vi "OdorSeq_Main.vi"() -> ()   [LabVIEW 2016]
uses:
  <vilib>/event_ctls.llb/eventvkey.ctl
  Odour_component_data_GLOBAL.vi
  <vilib>/Utility/xml.llb/Read From XML File(string).vi
  Odour_stimuli.vi
  Odour_sequences.vi
  Odour component similarity map.vi
  Odour_protocol.vi
panel:
  in  "Tab Control":T1(tab)=enum."Stimuli"
  in  "Clear protocol":bool
  in  "Protocol cluster":T2={"Sequence"=[], "Rel. requency"=[5.0], "Frequency"=[5.0], "Sequence interval"=200.0, "Rarest sequence "=200.0, "Randomization"=2} {"Randomization" items=["None", "Simple shuffle", "Block"]; "Rarest sequence" format="%#_g /h"; "Sequence interval" format="%#_g ms"; "Frequency" format="%.3f"}
  in  "Save protocol":bool
  in  "Protocol":path
  in  "Sequences":i32(listbox)=7
  out "Stimulus similarity labels 2":string[](array[string])=["S1", "S2", "S3", "UNC S-", "UNC S+", "COND 1", "COND 2", "BLANK"]
  out "Stimulus similarity labels 1":string[](array[string])=["S1", "S2", "S3", "UNC S-", "UNC S+", "COND 1", "COND 2", "BLANK"]
  out "Stimulus similarity":u32[][](array[colorbox])=[[16711680, 5132031, 395007, 5921535, 255, 987135, 7434751, 255], [5132031, 16711680, 16775930, 16770276, 16760510, 16738922, 16767963, 255], [395007, 16775930, 16711680, 11382271, 16742777, 16776701, 12434943, 255], [5921535, 16770276, 11382271, 16723245, 16382463, 16772075, 16765136, 255], [255, 16760510, 16742777, 16382463, 16731726, 16740978, 12763903, 255], [987135, 16738922, 16776701, 16772075, 16740978, 16711680, 15000831, 255], [7434751, 16767963, 12434943, 16765136, 12763903, 15000831, 16724273, 255], [255, 255, 255, 255, 255, 255, 255, 16711680]]
  in  "Counter  13-16":i32(listbox)=-1
  in  "Counter  9-12":i32(listbox)=-1
  in  "Counter  5-8":i32(listbox)=-1
  in  "Trashcan":i32(listbox)
  in  "Stimuli":i32(listbox)=6
  in  "Stimulus properties":T3={"Name"="COND 2", "Bottles "=-1, "Conc."=10.0, "Unit"=enum."ppm", "Duration"=100.0, "Add stimulus button"=FALSE, "Remove stimulus button "=FALSE} {"Duration" format="%#_g ms"}
  in  "Counter  1-4":i32(listbox)=-1
  out "Color Box 21":u32(colorbox)=3381759
  out "Color Box 12":u32(colorbox)=9868950
  out "Color Box 12":u32(colorbox)
  out "Color Box 20":u32(colorbox)=15725235
  out "Color Box 19":u32(colorbox)=13140224
  out "Color Box 18":u32(colorbox)=8388736
  out "Color Box 17":u32(colorbox)=32896
  out "Color Box 16":u32(colorbox)=16711935
  out "Color Box 15":u32(colorbox)=8405056
  out "Color Box 14":u32(colorbox)=65535
  out "Color Box 13":u32(colorbox)=8388863
  out "Color Box 12":u32(colorbox)=16743025
  out "Color Box 11":u32(colorbox)=15990570
  out "Color Box 10":u32(colorbox)=255
  out "Color Box 9":u32(colorbox)=6618880
  out "Color Box 8":u32(colorbox)=16711680
  in  "Monomolecular":i32(listbox)=6
  in  "Mixture":i32(listbox)=2
  in  "Blank":i32(listbox)=2
  out "Bottle chemical similarity":cluster{"MDS1":dbl[], "MDS2":dbl[]}[](graph)=[{"MDS1"=[0.3189845978019478, -0.5958047359661698], "MDS2"=[-0.19587325078604045, -0.0928400576289578]}, {"MDS1"=[0.10987962122155093, -0.2773805044856591], "MDS2"=[-0.2505324334838407, -0.2170165090375375]}, {"MDS1"=[-0.6430615610179795, -0.10227449366179224], "MDS2"=[0.40234001920080187, -0.5044648362602937]}, {"MDS1"=[-0.4431658258870894, -0.024797457597433275], "MDS2"=[-0.29472177172362407, -0.49208323822896083]}, {"MDS1"=[0.4573556658647923], "MDS2"=[0.5384723425872284]}, {"MDS1"=[-0.17173498215634928], "MDS2"=[0.4360302310022115]}, {"MDS1"=[0.47823511863963886], "MDS2"=[0.3906686856455658]}, {"MDS1"=[-0.3589435679497024], "MDS2"=[0.4668292977954712]}, {"MDS1"=[-0.14564084129683338], "MDS2"=[0.2496266112085214]}, {"MDS1"=[0.47341517045736714], "MDS2"=[0.47574696538692657]}, {"MDS1"=[-0.6803573756720218], "MDS2"=[-0.439251267008941]}]
  in  "Sequence properties":T4={"Name"="COMPLEX 2D+", "Trigger"=2, "Stimulus interval"=10.0, "Add sequence button"=FALSE, "Remove sequence button "=FALSE, "Stimuli "=0, "Reward condition"=0} {"Reward condition" items=["None", "Both / middle", "Left", "Right", "No-go"]; "Trigger" items=["None", "Sequence start", "Each stimulus"]; "Stimulus interval" format="%#_6g ms"}
  in  "Color Box 2":u32(colorbox)=255
  in  "Color Box":u32(colorbox)=16711680
  in  "DistanceMatrixColorBox":u32[][](array[colorbox])=[[13158600, 13158600, 13158600, 13158600, 13158600, 13158600, 13158600, 13158600, 13158600, 13158600, 13158600, 13158600, 13158600, 13158600, 13158600, 13158600], [13158600, 16736609, 10461183, 255, 16053503, 12369151, 255, 255, 16764879, 255, 16771818, 16773874, 15987711, 255, 11382271, 5526783], [13158600, 10461183, 16711680, 255, 16769762, 16727871, 255, 255, 11974399, 255, 16774645, 16119295, 12303359, 255, 16711680, 1645055], [13158600, 255, 255, 16711680, 255, 255, 16711680, 16711680, 255, 16711680, 255, 255, 255, 16711680, 255, 255], [13158600, 16053503, 16769762, 255, 16711680, 16757426, 255, 255, 15724543, 255, 16766164, 16736095, 16750230, 255, 16763851, 2566143], [13158600, 12369151, 16727871, 255, 16757426, 16711680, 255, 255, 11645439, 255, 16771304, 16766678, 15987711, 255, 16716563, 255], [13158600, 255, 255, 16711680, 255, 255, 16711680, 16711680, 255, 16711680, 255, 255, 255, 16711680, 255, 255], [13158600, 255, 255, 16711680, 255, 255, 16711680, 16711680, 255, 16711680, 255, 255, 255, 16711680, 255, 255], [13158600, 16764879, 11974399, 255, 15724543, 11645439, 255, 255, 16734810, 255, 16760767, 16772075, 12698111, 255, 11842815, 7697919], [13158600, 255, 255, 16711680, 255, 255, 16711680, 16711680, 255, 16711680, 255, 255, 255, 16711680, 255, 255], [13158600, 16771818, 16774645, 255, 16766164, 16771304, 255, 255, 16760767, 255, 16731469, 16763080, 14606079, 255, 16772075, 6645247], [13158600, 16773874, 16119295, 255, 16736095, 16766678, 255, 255, 16772075, 255, 16763080, 16711680, 16758454, 255, 16773103, 5724159], [13158600, 15987711, 12303359, 255, 16750230, 15987711, 255, 255, 12698111, 255, 14606079, 16758454, 16711680, 255, 14013951, 1776639], [13158600, 255, 255, 16711680, 255, 255, 16711680, 16711680, 255, 16711680, 255, 255, 255, 16711680, 255, 255], [13158600, 11382271, 16711680, 255, 16763851, 16716563, 255, 255, 11842815, 255, 16772075, 16773103, 14013951, 255, 16711680, 855551], [13158600, 5526783, 1645055, 255, 2566143, 255, 255, 255, 7697919, 255, 6645247, 5724159, 1776639, 255, 855551, 16711680]]
  out "Odour bottles":T5(array[cluster])=[[{"Mixture components"=[{"Name"="Acetophenone", "CID"=8174, "Volatility"=0.45}, {"Name"="Fenchone", "CID"=8635, "Volatility"=0.82}], "Name"="B1 (ME1)", "VPs"="6.4E-1 ± 41%", "Proportion"=[{"Numeric"=50.0}, {"Numeric"=50.0}], "Selected"=TRUE}, {"Mixture components"=[{"Name"="Methyl benzoate", "CID"=8103, "Volatility"=0.38}, {"Name"="Menthone", "CID"=8063, "Volatility"=0.28}], "Name"="B2 (ME2)", "VPs"="3.3E-1 ± 21%", "Proportion"=[{"Numeric"=50.0}, {"Numeric"=50.0}], "Selected"=FALSE}, {"Mixture components"=[{"Name"="Decanol", "CID"=460, "Volatility"=0.00851}], "Name"="B3 (C4f)", "VPs"="8.5E-3", "Proportion"=[{"Numeric"=100.0}], "Selected"=FALSE}, {"Mixture components"=[{"Name"="MINERAL OIL", "CID"=0, "Volatility"=0.0}], "Name"="B4 (Bl)", "VPs"="0.0E+0", "Proportion"=[{"Numeric"=100.0}], "Selected"=FALSE}], [{"Mixture components"=[{"Name"="Heptanoic acid ", "CID"=957, "Volatility"=0.0107}], "Name"="B5 (C3cA)", "VPs"="1.1E-2", "Proportion"=[{"Numeric"=100.0}], "Selected"=FALSE}, {"Mixture components"=[{"Name"="Octanol", "CID"=7439, "Volatility"=0.0794}], "Name"="B6 (C4cA)", "VPs"="7.9E-2", "Proportion"=[{"Numeric"=100.0}], "Selected"=FALSE}, {"Mixture components"=[{"Name"="MINERAL OIL", "CID"=0, "Volatility"=0.0}], "Name"="B7 (Bl)", "VPs"="0.0E+0", "Proportion"=[{"Numeric"=100.0}], "Selected"=FALSE}, {"Mixture components"=[{"Name"="MINERAL OIL", "CID"=0, "Volatility"=0.0}], "Name"="B8 (Bl)", "VPs"="0.0E+0", "Proportion"=[{"Numeric"=100.0}], "Selected"=FALSE}], [{"Mixture components"=[{"Name"="Geranyl acetate", "CID"=6985, "Volatility"=0.03}, {"Name"="Dimethylacetophenone", "CID"=7144, "Volatility"=0.063}], "Name"="B9 (MW1)", "VPs"="4.6E-2 ± 50%", "Proportion"=[{"Numeric"=50.0}, {"Numeric"=50.0}], "Selected"=FALSE}, {"Mixture components"=[{"Name"="MINERAL OIL", "CID"=0, "Volatility"=0.0}], "Name"="B10 (Bl)", "VPs"="0.0E+0", "Proportion"=[{"Numeric"=100.0}], "Selected"=FALSE}, {"Mixture components"=[{"Name"="Geraniol", "CID"=6405, "Volatility"=0.03}, {"Name"="Phenyl butanone", "CID"=7762, "Volatility"=0.1}], "Name"="B11 (MW2)", "VPs"="6.5E-2 ± 76%", "Proportion"=[{"Numeric"=50.0}, {"Numeric"=50.0}], "Selected"=FALSE}, {"Mixture components"=[{"Name"="Pentyl acetate", "CID"=12348, "Volatility"=3.5}], "Name"="B12 (C3f)", "VPs"="3.5E+0", "Proportion"=[{"Numeric"=100.0}], "Selected"=FALSE}], [{"Mixture components"=[{"Name"="Valeric acid", "CID"=8025, "Volatility"=0.196}], "Name"="B13 (C3cB)", "VPs"="2.0E-1", "Proportion"=[{"Numeric"=100.0}], "Selected"=FALSE}, {"Mixture components"=[{"Name"="MINERAL OIL", "CID"=0, "Volatility"=0.0}], "Name"="B14 (Bl)", "VPs"="0.0E+0", "Proportion"=[{"Numeric"=100.0}], "Selected"=FALSE}, {"Mixture components"=[{"Name"="Nonanol", "CID"=4133, "Volatility"=0.0227}], "Name"="B15 (C4cB)", "VPs"="2.3E-2", "Proportion"=[{"Numeric"=100.0}], "Selected"=FALSE}, {"Mixture components"=[{"Name"="Hydroxacetophenone", "CID"=7462, "Volatility"=0.0856}], "Name"="B16 (Ol)", "VPs"="8.6E-2", "Proportion"=[{"Numeric"=100.0}], "Selected"=FALSE}]] {"Proportion"."Numeric" format="%d%%"}
  in  "Odour chemicals":i32(listbox)=36
  out "Chemical similarity":cluster{"MDS1":dbl[], "MDS2":dbl[]}[](graph)=[{"MDS1"=[], "MDS2"=[]}, {"MDS1"=[396.3821953927539, -262.41250467128555, -231.36430031040578, 114.07056457899871, -29.645616081049297, 58.40307821935197, -213.3415540440491, 252.76854811630145, 114.59724760685786, 12.179301078164926, 213.71781772180816, 10.245213827208765, -317.9647981045101, 249.27752347690375, -296.4544615523987, -26.698853099282278, -303.9529163482059, -23.502678410472118, -79.59753085274536, -76.44304440140283, -294.6567457719659, 112.29360419618213, -273.35122450752266, -294.76791641311274, -269.340230018179, -191.41524828002733, 251.79971870928094, 205.2249479165084, 515.3849497534994, -126.91499848915312, -152.14035558594634, -152.674775911407, -208.04948323720893, -111.19908951088753, -235.0545852465996, -236.20336645538308, -165.64242245257407, 110.87943807753645, -159.5151592759888, -148.46677914865614, 197.2464957982167, -232.541000525234, -187.82662250571298, -122.94463556800827, -191.8219737813257, 180.22600495656366, 51.353048668431704, -158.52742292807153, 266.82605746771884, -244.97562606669857, 207.17154717294608, -35.65469956598489, 256.9928159423369, -246.95298712232488, 143.47309690220376, -252.7110045881726, 150.23211981471368, 21.156685543603103, 179.59046460245207, -210.9178904519634, 281.28159545024744, 47.27018090750722, 185.8537823396016, -120.17144764398293, 119.41963149938562, -58.24361669961045, 17.20580648407221, -19.733594212360888, -2.8949993967070853, 14.89385579391006, 204.32713615045907, 31.18693554024182, 236.49773623152166, 37.27700380001177, 51.170561159934444, 297.4652966197888, 258.01381231117176, 93.81548252939837, 98.13934241781413, 233.76965217524653, 147.75453833538387, 339.8533239503384, -inf], "MDS2"=[-294.1625463085245, 75.06909387065261, 203.83961706757722, -243.76771476212969, -281.62183144789145, -228.79990905087422, 296.65536658552134, -250.34883594312083, -96.63812347643292, -164.80443024342875, -327.1617713637844, -277.3638544350568, -43.831335920252606, -213.31743810727397, 107.12891384196561, -87.93548942481429, 9.54512145075226, -253.81154308548392, -324.2771585204367, -273.6441237325548, 122.4114919562466, 39.85287306331019, -42.263086129371295, 191.0620800004279, -95.83774156123017, 142.3631394442883, -161.91563269564605, -308.24507263086724, -68.17744072149127, 102.91867516437394, -143.60083658864872, 243.13326408951488, -158.23331010430897, 208.56819115230442, -26.650521263465556, -104.36500693122969, -73.95049456240373, 170.98018005743705, 8.436616623045376, -213.0788157505672, -238.619079383165, 130.6588221918013, 101.29743735356698, 191.9015477463772, 189.9450263215761, 104.35598527492789, -178.40967800200966, -249.66981496564088, 13.479384089782926, -207.08642326769737, -174.93797693620664, 270.2139888611614, -68.61957940549138, -204.5270138088883, -211.27776405264314, -217.6654971930947, 221.1580180551867, -115.32895882976128, -56.04022976112759, 38.88407874545689, 102.71121558509061, -66.65120683967478, 288.33901581648973, 295.9933132570569, -28.685096728203234, 130.29205926060382, -8.697992950423888, 18.78620227069331, 37.62756232510908, 133.32677712624545, 160.28624069412643, 86.77073317156534, 93.65722557836662, 217.8007894783545, 191.40195381349582, 315.17787277483853, 146.47302969001294, 259.6981542624837, 398.7044129905194, 190.396254515234, 281.1287978570423, 251.5898534107341, -inf]}]
  in  "Distance metric":string(combo)="canberra_all"
  # "1"
  # "2"
  # "3"
  # "4"
  # "5"
  # "6"
  # "7"
  # "8"
  # "9"
  # "10"
  # "11"
  # "12"
  # "13"
  # "14"
  # "15"
  # "16"
  # "1"
  # "2"
  # "3"
  # "4"
  # "Similar"
  # "5"
  # "6"
  # "Different"
  # "7"
  # "8"
  # "9"
  # "10"
  # "11"
  # "12"
  # "13"
  # "14"
  # "15"
  # "16"
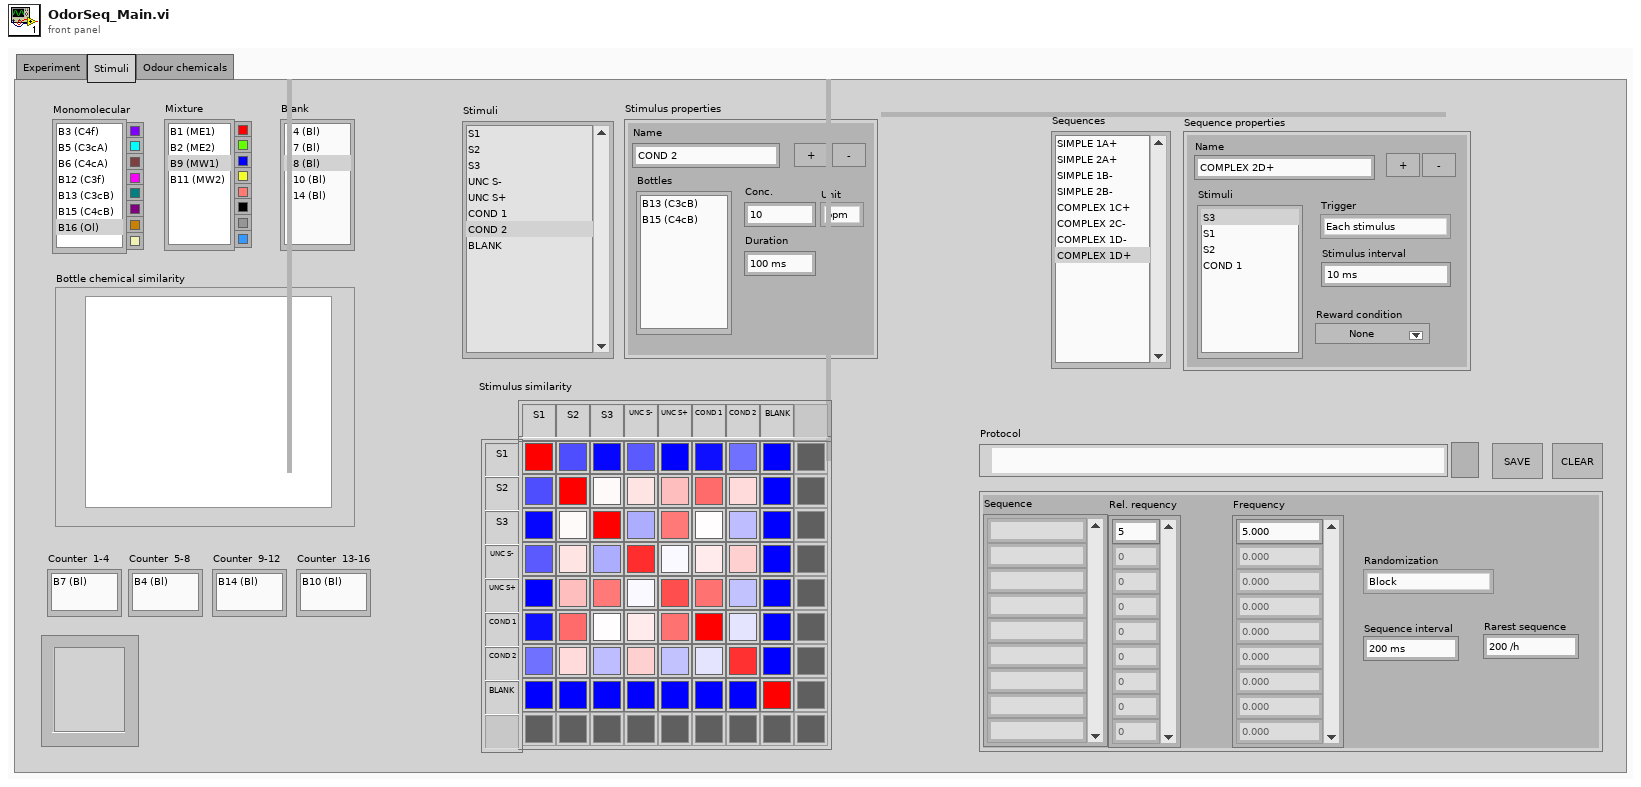
[diagram p1: front panel]
types:
  T1 = enum32{"Experiment", "Stimuli", "Odour chemicals"}
  T2 = cluster{"Sequence":string[], "Rel. requency":dbl[], "Frequency":dbl[], "Sequence interval":dbl, "Rarest sequence ":dbl, "Randomization":u16}
  T3 = cluster{"Name":string, "Bottles ":i32, "Conc.":dbl, "Unit":enum16{"%", "ppm"}, "Duration":dbl, "Add stimulus button":bool, "Remove stimulus button ":bool}
  T4 = cluster{"Name":string, "Trigger":u16, "Stimulus interval":dbl, "Add sequence button":bool, "Remove sequence button ":bool, "Stimuli ":i32, "Reward condition":u16}
  T5 = cluster{"Mixture components":cluster{"Name":string, "CID":i32, "Volatility":dbl}[], "Name":string, "VPs":string, "Proportion":cluster{"Numeric":dbl}[], "Selected":bool}[][]
  T6 = cluster{"names":string[], "CID":i32[], "volatility":dbl[], "2D map":dbl[][], "distance matrix":dbl[][]}
  T7 = cluster{"Name":string, "Bottles":i32[], "Conc.":dbl, "Unit":enum16{"%", "ppm"}, "Frequency":dbl}[]
  T8 = cluster{"Name":string, "Trigger":u16, "Stimulus interval":dbl, "Stimuli":i32[], "Reward condition":u16}[]
  T9 = cluster{"Name":string, "Bottles":i32[], "Conc.":dbl, "Unit":enum16{"%", "ppm"}, "Frequency":dbl}
  T10 = cluster{"Name":string, "Trigger":u16, "Stimulus interval":dbl, "Stimuli":i32[], "Reward condition":u16}
  T11 = typedef "eventvkey.ctl" = enum16{"ASCII", "Enter", "Return", "Shift", "Ctrl", "Alt", "Cmd", "Opt", "Caps", "NumLock", "Clear", "Break", "Up", "Down", "Left", "Right", "Insert", "Delete", "Home", "End", "PageUp", "PageDown", "Escape", "Help", "Pause", "ScrollLock", "F1", "F2", "F3", "F4", "F5", "F6", "F7", "F8", "F9", "F10", "F11", "F12", "F13", "F14", "F15", "F16", "F17", "F18", "F19", "F20", "F21", "F22", "F23", "F24", "Play", "VolumeUp", "VolumeDown", "Mute", "Two Byte Char"}
  T12 = cluster{"names":string[], "CID":i32[], "Vapour pressure":dbl[], "2D map":dbl[][], "distance matrix":dbl[][]}
  T13 = cluster{"Mixture components":cluster{"Name":string, "CID":i32, "Volatility":dbl}[], "Name":string, "VPs":string, "Proportion":cluster{"Numeric":dbl}[], "Selected":bool}[]
  T14 = cluster{"Name":string, "CID":i32, "Volatility":dbl}[]
  T15 = typedef "LVPoint32TypeDef.ctl" = cluster{"Horizontal":i32, "Vertical":i32}
  T16 = typedef "LVBoundsTypeDef.ctl" = cluster{"Width":u32, "Height":u32}
  T17 = typedef "LVPositionTypeDef.ctl" = cluster{"Left":i32, "Top":i32}
  T18 = cluster{"Mixture components":cluster{"Name":string, "CID":i32, "Volatility":dbl}[], "Name":string, "VPs":string, "Proportion":cluster{"Numeric":dbl}[], "Selected":bool}
  T19 = cluster{"Name":string, "Bottles":i32[], "Conc.":dbl, "Unit":enum16{"%", "ppm"}, "Duration":dbl}[]
  T20 = cluster{"Name":string, "Bottles":i32[], "Conc.":dbl, "Unit":enum16{"%", "ppm"}, "Duration":dbl}
  T21 = cluster{"data name":string, "drag data":variant}[]
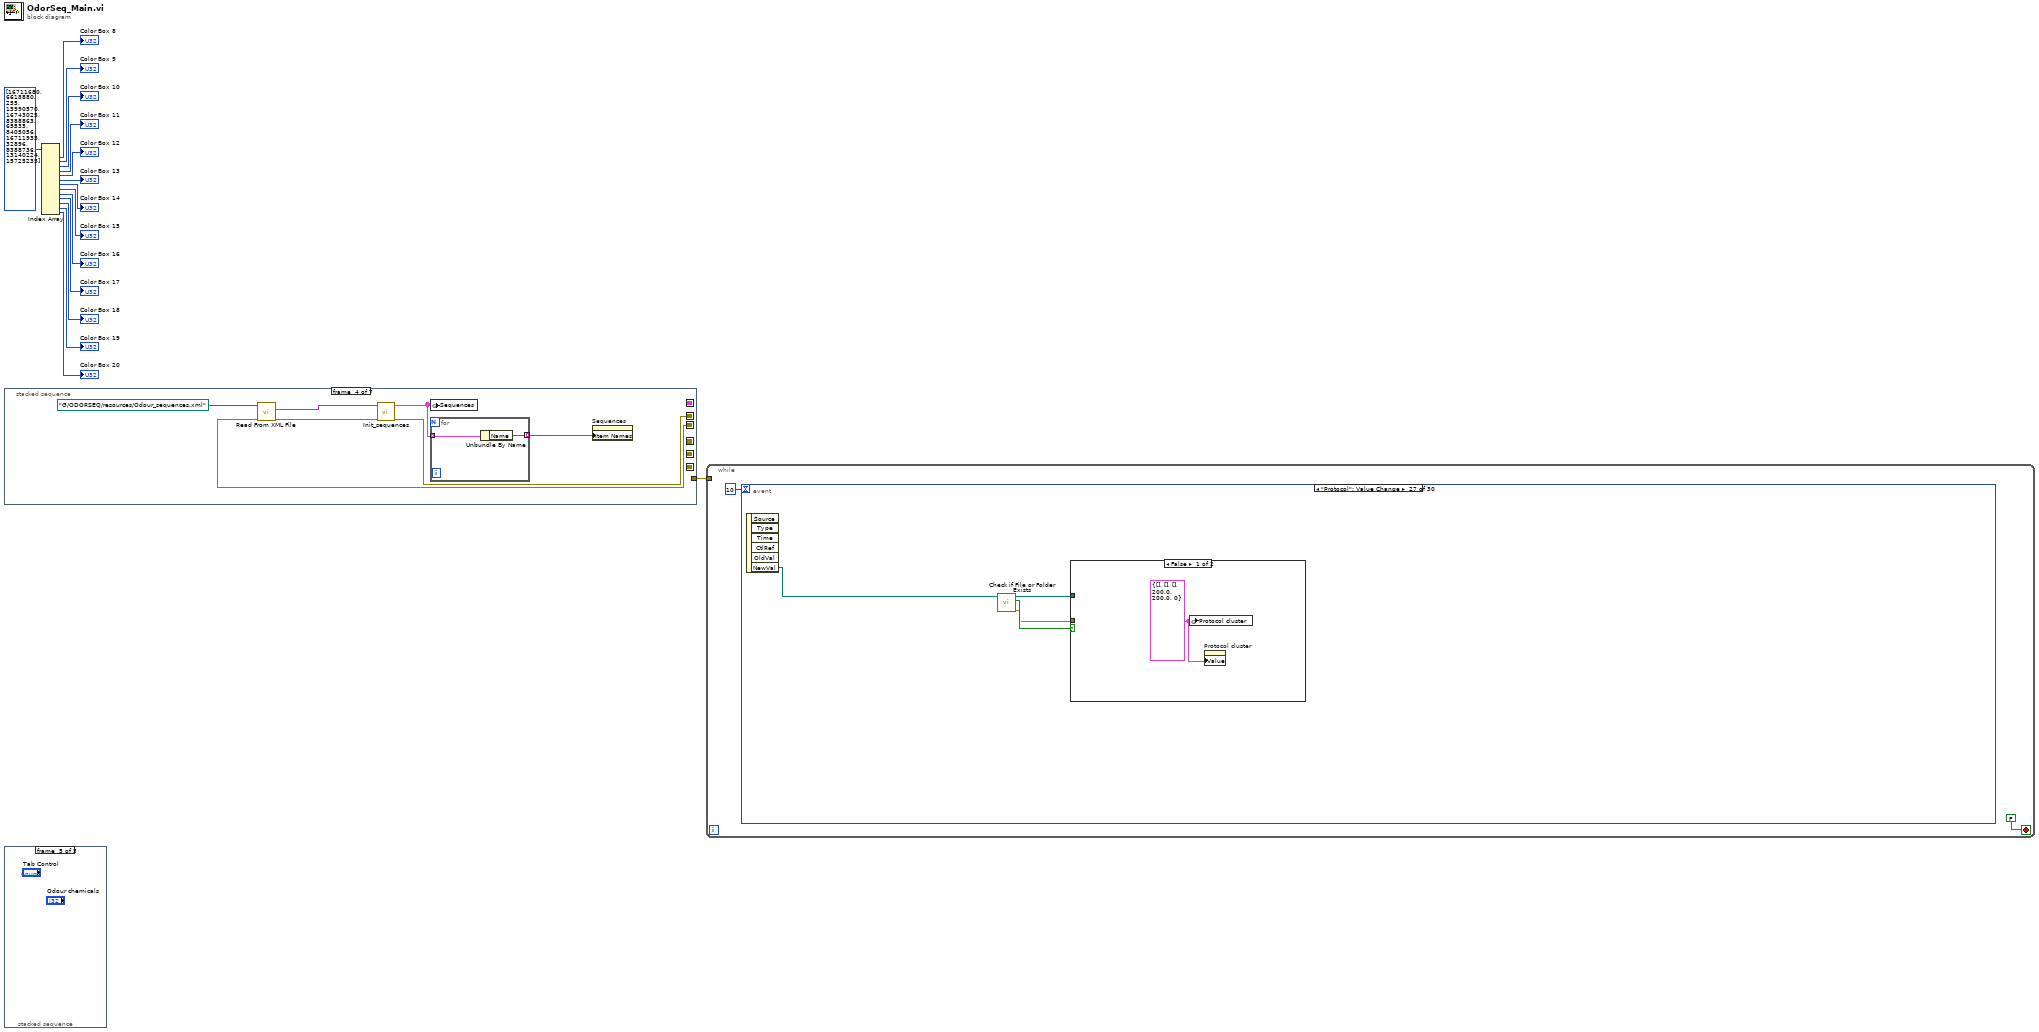
[diagram p0: block diagram]
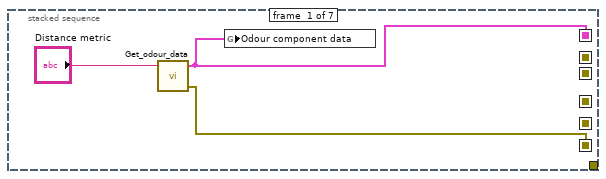
[diagram p2: hidden frame]
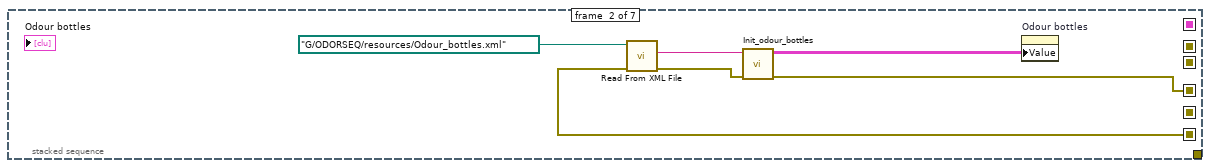
[diagram p3: hidden frame]
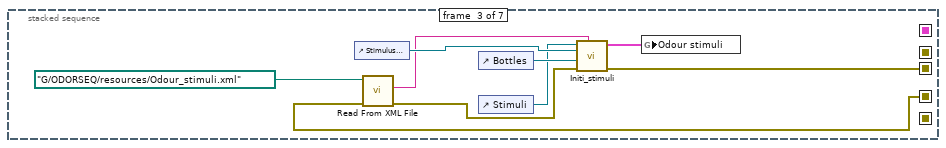
[diagram p4: hidden frame]
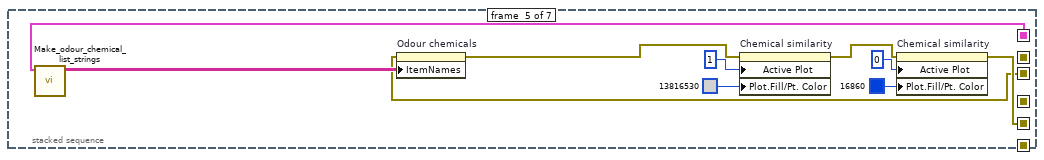
[diagram p5: hidden frame]
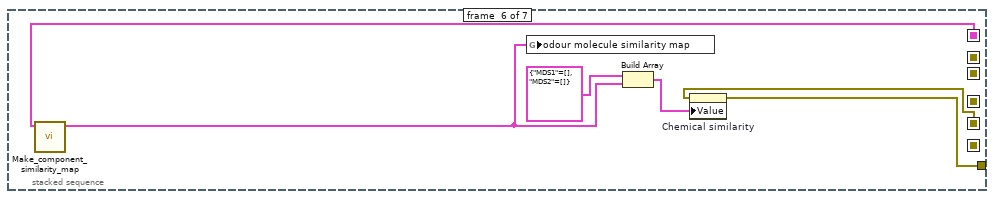
[diagram p6: hidden frame]
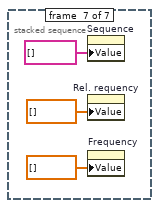
[diagram p7: hidden frame]
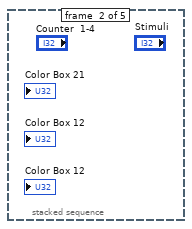
[diagram p9: hidden frame]
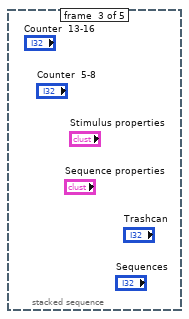
[diagram p10: hidden frame]
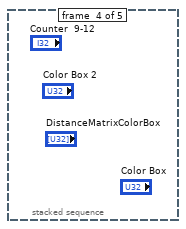
[diagram p11: hidden frame]
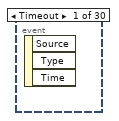
[diagram p12: hidden frame]
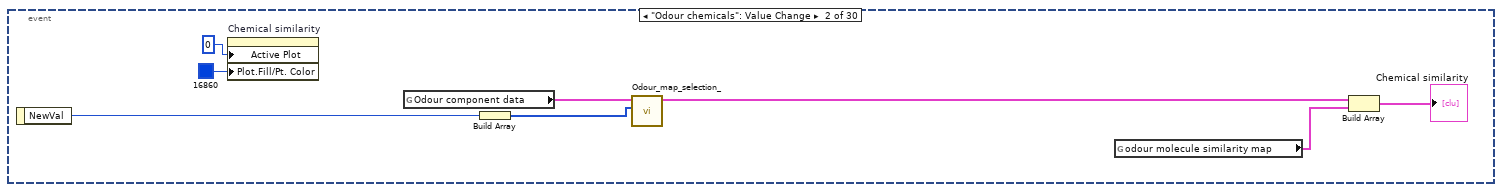
[diagram p13: hidden frame]
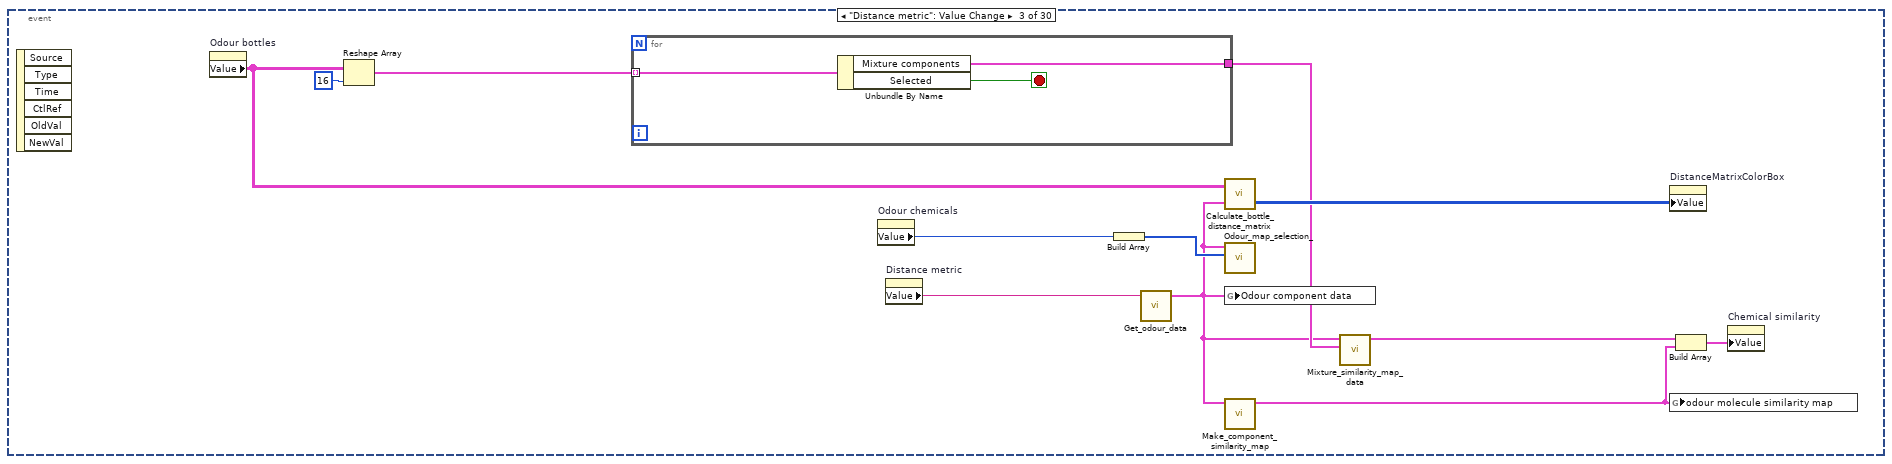
[diagram p14: hidden frame]
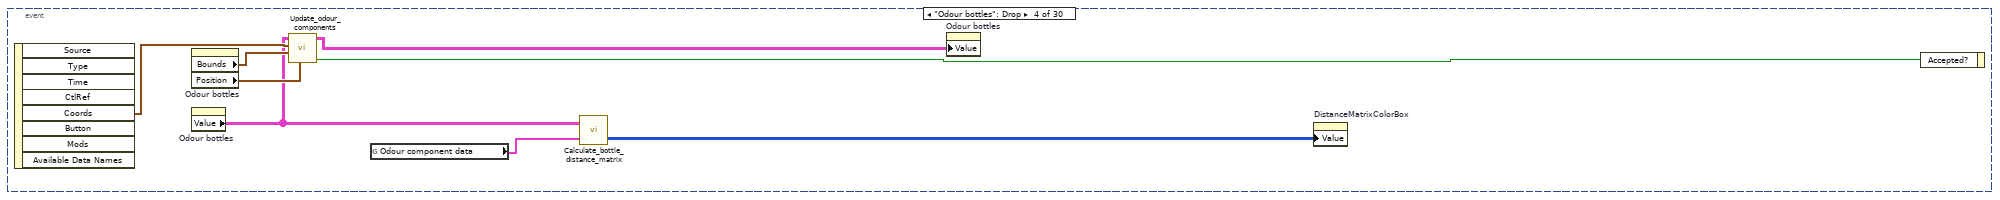
[diagram p15: hidden frame]
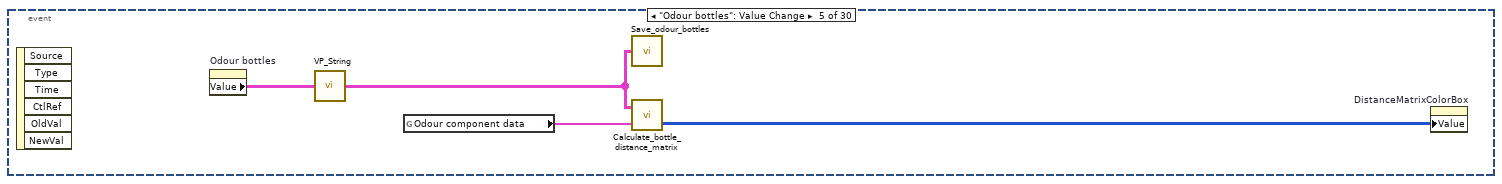
[diagram p16: hidden frame]
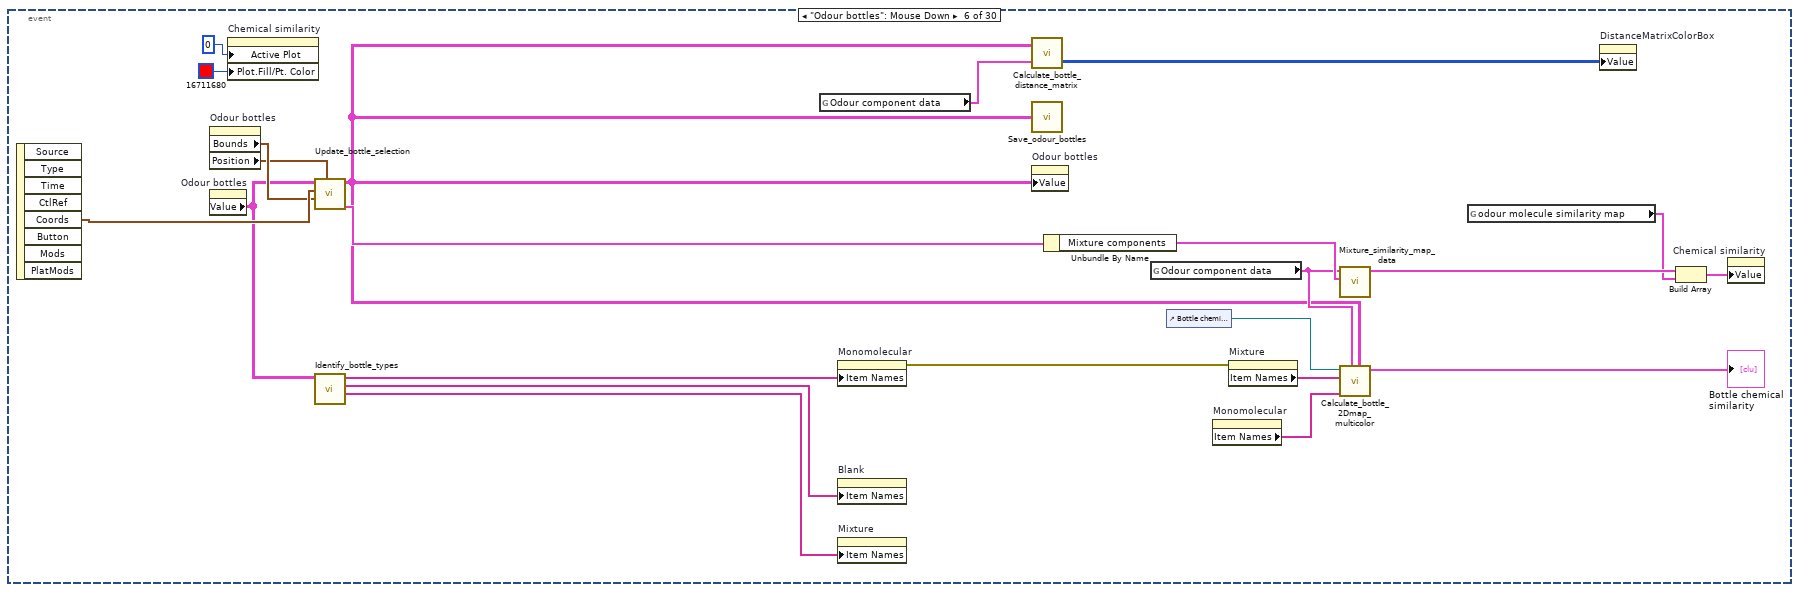
[diagram p17: hidden frame]
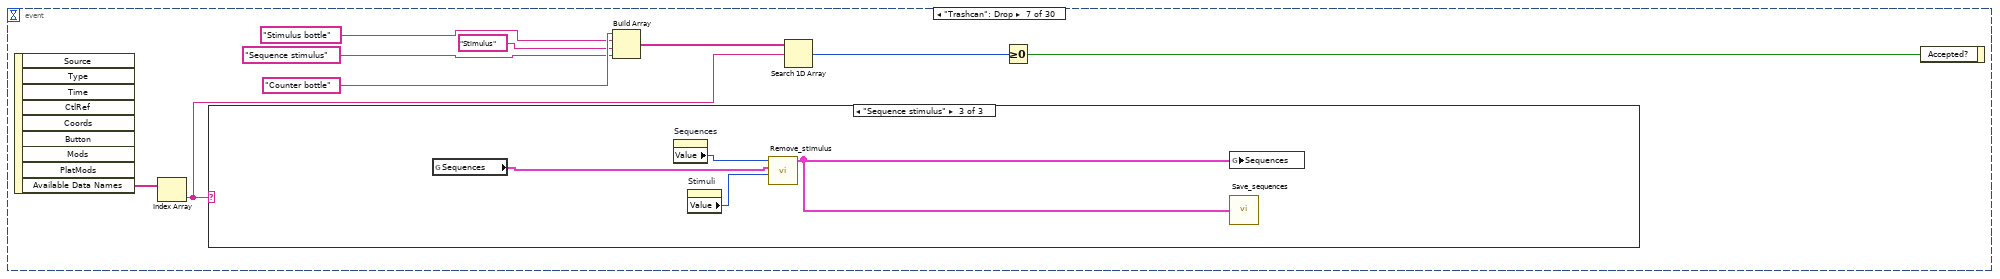
[diagram p18: hidden frame]
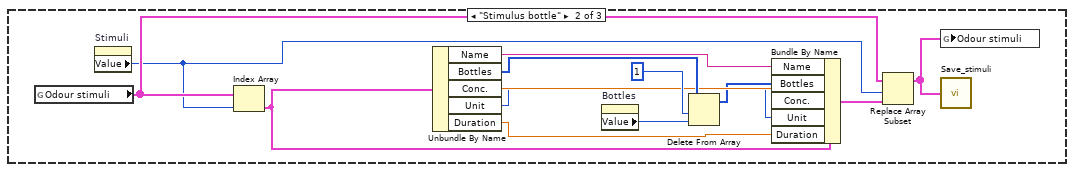
[diagram p20: hidden frame]
diagram:
  n1 = stacked-sequence {
    seq-local: [w16 _ _ _ _ _ _] -> [_ _ _ _ w44 w55 _]
    seq-local: [w17 _ _ _ _ _ _] -> [_ w21 _ _ _ _ _]
    seq-local: [_ w20 _ _ _ _ _] -> [_ _ w27 _ _ _ _]
    seq-local: [_ _ w26 _ _ _ _] -> [_ _ _ w40 w43 _ _]
    seq-local: [_ _ _ _ w45 _ _] -> [_ _ _ _ _ w54 _]
    seq-local: [_ _ _ w36 _ _ _] -> [_ _ _ _ _ _ _]
    tunnel: [_ _ _ _ _ w53 _] -> w1
    frame #0 {
      n2 = call "Get_odour_data.vi"("Distance metric"="Distance metric") -> ("error out"=w17:errorcluster, "Odour component data"=w16:T6)  [unwired: 3 in]
      n3 = global write "Odour_component_data_GLOBAL.vi" "Odour component data"(w16) -> ()
    }
    frame #1 {
      n4 = call-poly <vilib>:"Read From XML File.vi"("error in (no error)"=w21, "XML File Path"=path "G:/ODORSEQ/resources/Odour_bottles.xml") -> ("error out"=w24:errorcluster, "XML Elements"=w23:string)  [unwired: 7 in, 1 out]
      n5 = call "Init_odour_bottles.vi"("error in (no error)"=w24, "XML Elements"=w23) -> ("error IO"=w20:errorcluster, "Array"=w19:T5)  [unwired: 8 in]
      n6 = property on="Odour bottles" class="Arr (strict)"("Value"=w19) -> ()  [unwired: 2 in, 2 out]
    }
    frame #2 {
      n7 = control-ref of="Stimulus properties"() -> (w32:refnum<vi>)
      n8 = call-poly <vilib>:"Read From XML File.vi"("error in (no error)"=w27, "XML File Path"=path "G:/ODORSEQ/resources/Odour_stimuli.xml") -> ("error out"=w28:errorcluster, "XML Elements"=w29:string)  [unwired: 7 in, 1 out]
      n9 = control-ref of="Bottles"() -> (w33:refnum<vi>)
      n10 = control-ref of="Stimuli"() -> (w31:refnum<vi>)
      n11 = call "Initi_stimuli.vi"("XML Elements"=w29, "error in (no error)"=w28, "LstBox Refnum in"=w33, "Clust Refnum"=w32, "ListBox in"=w31) -> ("error IO"=w26:errorcluster, "Array"=w25:T7)  [unwired: 5 in]
      n12 = global write "Odour_stimuli.vi" "Odour stimuli"(w25) -> ()
    }
    frame #3 {
      n13 = call-poly <vilib>:"Read From XML File.vi"("error in (no error)"=w40, "XML File Path"=path "G:/ODORSEQ/resources/Odour_sequences.xml") -> ("error out"=w37:errorcluster, "XML Elements"=w38:string)  [unwired: 7 in, 1 out]
      n14 = call "Init_sequences.vi"("error in (no error)"=w37, "XML Elements"=w38) -> ("error IO"=w36:errorcluster, "Sequences"=w34:T8)  [unwired: 8 in]
      n15 = global write "Odour_sequences.vi" "Sequences"(w34) -> ()
      n16 = for {
        tunnel: [w42] -> w35 mode=indexing
        tunnel: w34 -> [w41] mode=indexing
        n17 = Unbundle By Name(w41) -> ("Name"=w42:string)
      }
      n18 = property on="Sequences" class="LstBox (strict)"("Item Names"=w35) -> ()  [unwired: 2 in, 2 out]
    }
    frame #4 {
      n19 = call "Make_odour_chemical_list_strings.vi"("Odour component data"=w44) -> ("Array"=w51:string[][])  [unwired: 10 in]
      n20 = property on="Odour chemicals" class="MCListbox (strict)"(error in=w43, "ItemNames"=w51) -> (error out=w52:errorcluster)  [unwired: 1 in, 1 out]
      n21 = property on="Chemical similarity" class="XYGraph (strict)"(error in=w52, "Active Plot"=u32 1, "Plot.Fill/Pt. Color"=u32 13816530) -> (error out=w47:errorcluster)  [unwired: 1 in, 1 out]
      n22 = property on="Chemical similarity" class="XYGraph (strict)"(error in=w47, "Active Plot"=u32 0 ("Plot.Fill/Point Color"), "Plot.Fill/Pt. Color"=u32 16860) -> (error out=w45:errorcluster)  [unwired: 1 in, 1 out]
    }
    frame #5 {
      n23 = call "Make_component_similarity_map.vi"("Odour component data"=w55) -> ("input cluster"=w56:cluster{"MDS1":dbl[], "MDS2":dbl[]})  [unwired: 10 in]
      n24 = global write "Odour component similarity map.vi" "odour molecule similarity map"(w56) -> ()
      n25 = Build Array(cluster{"MDS1":dbl[], "MDS2":dbl[]} {"MDS1"=[], "MDS2"=[]} ("element"), w56) -> (w57:cluster{"MDS1":dbl[], "MDS2":dbl[]}[])
      n26 = property on="Chemical similarity" class="XYGraph (strict)"(error in=w54, "Value"=w57) -> (error out=w53:errorcluster)  [unwired: 1 in, 1 out]
    }
    frame #6 {
      n27 = property on="Sequence" class="Arr (strict)"("Value"=string[] [] ("Item Names")) -> ()  [unwired: 2 in, 2 out]
      n28 = property on="Rel. requency" class="Arr (strict)"("Value"=dbl[] [] ("Rel. requency")) -> ()  [unwired: 2 in, 2 out]
      n29 = property on="Frequency" class="Arr (strict)"("Value"=dbl[] [] ("Frequency")) -> ()  [unwired: 2 in, 2 out]
    }
  }
  n30 = stacked-sequence {
    frame #0 {
    }
    frame #1 {
    }
    frame #2 {
    }
    frame #3 {
    }
    frame #4 {
    }
  }
  n31 = Index Array(array=u32[] [16711680, 6618880, 255, 15990570, 16743025, 8388863, 65535, 8405056, 16711935, 32896, 8388736, 13140224, 15725235]) -> (element #1=→"Color Box 8":u32, element #2=→"Color Box 9":u32, element #3=→"Color Box 10":u32, element #4=→"Color Box 11":u32, element #5=→"Color Box 12":u32, element #6=→"Color Box 13":u32, element #7=→"Color Box 14":u32, element #8=→"Color Box 15":u32, element #9=→"Color Box 16":u32, element #10=→"Color Box 17":u32, element #11=→"Color Box 18":u32, element #12=→"Color Box 19":u32, element #13=→"Color Box 20":u32)  [unwired: 13 in]
  n32 = while {
    tunnel: w1 -> [_]
    stop <- FALSE stop-if-true
    n33 = event shown="[26] \"Protocol\": Value Change" {
      selector: _ -> [_ _ _ _ _ _ _ _ _ _ _ _ _ _ _ _ _ _ _ _ _ _ _ _ _ _ _ _ _ _]
      dyn-events: _ -> [_ _ _ _ _ _ _ _ _ _ _ _ _ _ _ _ _ _ _ _ _ _ _ _ _ _ _ _ _ _]
      timeout: 10 -> [_ _ _ _ _ _ _ _ _ _ _ _ _ _ _ _ _ _ _ _ _ _ _ _ _ _ _ _ _ _]
      event Timeout {
        n34 = event-data() -> ()  [unwired: 1 in, 3 out]
      }
      event "Odour chemicals": Value Change {
        n35 = event-data() -> ("NewVal"=w71:i32)  [unwired: 1 in]
        n36 = property on="Chemical similarity" class="XYGraph (strict)"("Active Plot"=u32 0 ("Plot.Fill/Point Color"), "Plot.Fill/Pt. Color"=u32 16860) -> ()  [unwired: 2 in, 2 out]
        n37 = global read "Odour_component_data_GLOBAL.vi" "Odour component data"() -> (w66:T12)
        n38 = Build Array(w71) -> (w65:i32[])
        n39 = call "Odour_map_selection_.vi"("Array"=w65, "Odour component data"=w66) -> ("input cluster"=w69:cluster{"MDS1":dbl[], "MDS2":dbl[]})  [unwired: 9 in]
        n40 = global read "Odour component similarity map.vi" "odour molecule similarity map"() -> (w64:cluster{"MDS1":dbl[], "MDS2":dbl[]})
        n41 = Build Array(w69, w64) -> (→"Chemical similarity":cluster{"MDS1":dbl[], "MDS2":dbl[]}[])
      }
      event "Distance metric": Value Change {
        n42 = event-data() -> ()  [unwired: 1 in, 6 out]
        n43 = property on="Odour bottles" class="Arr (strict)"() -> ("Value"=w77:T5)  [unwired: 2 in, 2 out]
        n44 = Reshape Array(w77, 16 ("dimension size")) -> (w76:T13)
        n45 = for {
          tunnel: w76 -> [w86] mode=indexing
          tunnel: [w84] -> w74
          stop <- w85 stop-if-true
          n46 = Unbundle By Name(w86) -> ("Mixture components"=w84:T14, "Selected"=w85:bool)
        }
        n47 = property on="Odour chemicals" class="MCListbox (strict)"() -> ("Value"=w81:i32)  [unwired: 2 in, 2 out]
        n48 = property on="Distance metric" class="CmbBox"() -> ("Value"=w80:string)  [unwired: 2 in, 2 out]
        n49 = Build Array(w81) -> (w83:i32[])
        n50 = call "Get_odour_data.vi"("Distance metric"=w80) -> ("Odour component data"=w72:T6)  [unwired: 3 in, 1 out]
        n51 = call "Calculate_bottle_distance_matrix.vi"("Odour component data"=w72, "Odour bottles"=w77) -> ("Colour grid"=w78:u32[][])  [unwired: 1 in]
        n52 = call "Odour_map_selection_.vi"("Array"=w83, "Odour component data"=w72) -> ()  [unwired: 9 in, 1 out]
        n53 = global write "Odour_component_data_GLOBAL.vi" "Odour component data"(w72) -> ()
        n54 = call "Make_component_similarity_map.vi"("Odour component data"=w72) -> ("input cluster"=w79:cluster{"MDS1":dbl[], "MDS2":dbl[]})  [unwired: 10 in]
        n55 = call "Mixture_similarity_map_data.vi"("Mixture components"=w74, "Odour component data"=w72) -> ("input cluster"=w73:cluster{"MDS1":dbl[], "MDS2":dbl[]})  [unwired: 9 in]
        n56 = property on="DistanceMatrixColorBox" class="Arr (strict)"("Value"=w78) -> ()  [unwired: 2 in, 2 out]
        n57 = global write "Odour component similarity map.vi" "odour molecule similarity map"(w79) -> ()
        n58 = Build Array(w73, w79) -> (w82:cluster{"MDS1":dbl[], "MDS2":dbl[]}[])
        n59 = property on="Chemical similarity" class="XYGraph (strict)"("Value"=w82) -> ()  [unwired: 2 in, 2 out]
      }
      event "Odour bottles": Drop {
        n60 = event-data() -> ("Coords"=w94:T15)  [unwired: 1 in, 7 out]
        n61 = property on="Odour bottles" class="Arr (strict)"() -> ("Bounds"=w92:T16, "Position"=w93:T17)  [unwired: 2 in, 2 out]
        n62 = property on="Odour bottles" class="Arr (strict)"() -> ("Value"=w88:T5)  [unwired: 2 in, 2 out]
        n63 = call "Update_odour_components.vi"("Position"=w93, "Bounds"=w92, "Coords"=w94, "Odour bottles in"=w88) -> ("accept"=w91:bool, "Odou bottle out"=w89:T5)  [unwired: 6 in]
        n64 = global read "Odour_component_data_GLOBAL.vi" "Odour component data"() -> (w87:T12)
        n65 = call "Calculate_bottle_distance_matrix.vi"("Odour component data"=w87, "Odour bottles"=w88) -> ("Colour grid"=w90:u32[][])  [unwired: 1 in]
        n66 = property on="Odour bottles" class="Arr (strict)"("Value"=w89) -> ()  [unwired: 2 in, 2 out]
        n67 = property on="DistanceMatrixColorBox" class="Arr (strict)"("Value"=w90) -> ()  [unwired: 2 in, 2 out]
        n68 = event-data("Accepted?"=w91) -> ()  [unwired: 1 in, 1 out]
      }
      event "Odour bottles": Value Change {
        n69 = event-data() -> ()  [unwired: 1 in, 6 out]
        n70 = property on="Odour bottles" class="Arr (strict)"() -> ("Value"=w97:T5)  [unwired: 2 in, 2 out]
        n71 = call "VP_String.vi"("Odour bottles"=w97) -> ("Odour bottles 2"=w95:T5)
        n72 = global read "Odour_component_data_GLOBAL.vi" "Odour component data"() -> (w96:T12)
        n73 = call "Save_odour_bottles.vi"("Odour bottles"=w95) -> ()
        n74 = call "Calculate_bottle_distance_matrix.vi"("Odour component data"=w96, "Odour bottles"=w95) -> ("Colour grid"=w98:u32[][])  [unwired: 1 in]
        n75 = property on="DistanceMatrixColorBox" class="Arr (strict)"("Value"=w98) -> ()  [unwired: 2 in, 2 out]
      }
      event "Odour bottles": Mouse Down {
        n76 = event-data() -> ("Coords"=w121:T15)  [unwired: 1 in, 7 out]
        n77 = property on="Odour bottles" class="Arr (strict)"() -> ("Bounds"=w120:T16, "Position"=w119:T17)  [unwired: 2 in, 2 out]
        n78 = property on="Odour bottles" class="Arr (strict)"() -> ("Value"=w106:T5)  [unwired: 2 in, 2 out]
        n79 = property on="Chemical similarity" class="XYGraph (strict)"("Active Plot"=u32 0 ("Plot.Fill/Point Color"), "Plot.Fill/Pt. Color"=u32 16711680) -> ()  [unwired: 2 in, 2 out]
        n80 = call "Update_bottle_selection.vi"("Position"=w119, "Bounds"=w120, "Coords"=w121, "Odour bottles in"=w106) -> ("selected bottle"=w105:T18, "Odour bottles out"=w99:T5)  [unwired: 4 in]
        n81 = call "Identify_bottle_types.vi"("Odour bottles"=w106) -> ("Mixture bottles"=w112:string[], "Blank bottles"=w114:string[], "Monomolecular bottles"=w113:string[])  [unwired: 8 in]
        n82 = global read "Odour_component_data_GLOBAL.vi" "Odour component data"() -> (w100:T12)
        n83 = property on="Monomolecular" class="LstBox (strict)"("Item Names"=w113) -> (error out=w103:errorcluster)  [unwired: 2 in, 1 out]
        n84 = property on="Blank" class="LstBox (strict)"("Item Names"=w114) -> ()  [unwired: 2 in, 2 out]
        n85 = property on="Mixture" class="LstBox (strict)"("Item Names"=w112) -> ()  [unwired: 2 in, 2 out]
        n86 = call "Calculate_bottle_distance_matrix.vi"("Odour component data"=w100, "Odour bottles"=w99) -> ("Colour grid"=w101:u32[][])  [unwired: 1 in]
        n87 = call "Save_odour_bottles.vi"("Odour bottles"=w99) -> ()
        n88 = property on="Odour bottles" class="Arr (strict)"("Value"=w99) -> ()  [unwired: 2 in, 2 out]
        n89 = Unbundle By Name(w105) -> ("Mixture components"=w104:T14)
        n90 = global read "Odour_component_data_GLOBAL.vi" "Odour component data"() -> (w102:T12)
        n91 = control-ref of="Bottle chemical similarity"() -> (w109:refnum<vi>)
        n92 = property on="Monomolecular" class="LstBox (strict)"() -> ("Item Names"=w108:string[])  [unwired: 2 in, 2 out]
        n93 = property on="Mixture" class="LstBox (strict)"(error in=w103) -> ("Item Names"=w111:string[])  [unwired: 1 in, 2 out]
        n94 = call "Mixture_similarity_map_data.vi"("Mixture components"=w104, "Odour component data"=w102) -> ("input cluster"=w118:cluster{"MDS1":dbl[], "MDS2":dbl[]})  [unwired: 9 in]
        n95 = call "Calculate_bottle_2Dmap_multicolor.vi"("XYGraph in"=w109, "Mixture"=w111, "Monomolecular"=w108, "Odour component data"=w102, "Odour bottles in"=w99) -> ("appended array"=→"Bottle chemical similarity":cluster{"MDS1":dbl[], "MDS2":dbl[]}[])  [unwired: 5 in]
        n96 = global read "Odour component similarity map.vi" "odour molecule similarity map"() -> (w107:cluster{"MDS1":dbl[], "MDS2":dbl[]})
        n97 = property on="DistanceMatrixColorBox" class="Arr (strict)"("Value"=w101) -> ()  [unwired: 2 in, 2 out]
        n98 = Build Array(w118, w107) -> (w117:cluster{"MDS1":dbl[], "MDS2":dbl[]}[])
        n99 = property on="Chemical similarity" class="XYGraph (strict)"("Value"=w117) -> ()  [unwired: 2 in, 2 out]
      }
      event "Trashcan": Drop {
        n100 = event-data() -> ("Available Data Names"=w123:string[])  [unwired: 1 in, 8 out]
        n101 = Index Array(array=w123) -> (element=w124:string)  [unwired: 1 in]
        n102 = case shown="\"Sequence stimulus\"" w124 {
          frame "0", Default {
          }
          frame "Stimulus bottle" {
            n103 = global read "Odour_stimuli.vi" "Odour stimuli"() -> (w143:T19)
            n104 = property on="Stimuli" class="LstBox (strict)"() -> ("Value"=w134:i32)  [unwired: 2 in, 2 out]
            n105 = Index Array(array=w143, index=w134) -> (element=w135:T20)
            n106 = Unbundle By Name(w135) -> ("Name"=w139:string, "Bottles"=w142:i32[], "Conc."=w138:dbl, "Unit"=w137:enum16{"%", "ppm"}, "Duration"=w136:dbl)
            n107 = property on="Bottles" class="LstBox (strict)"() -> ("Value"=w141:i32)  [unwired: 2 in, 2 out]
            n108 = Delete From Array(array=w142, length=1, index=w141) -> (array with subset deleted=w132:i32[])  [unwired: 1 out]
            n109 = Bundle By Name(cluster=w135, "Name"=w139, "Bottles"=w132, "Conc."=w138, "Unit"=w137, "Duration"=w136) -> (w133:T20)
            n110 = Replace Array Subset(array=w143, new element=w133, index=w134) -> (w131:T19)
            n111 = global write "Odour_stimuli.vi" "Odour stimuli"(w131) -> ()
            n112 = call "Save_stimuli.vi"("Array"=w131) -> ()
          }
          frame "Sequence stimulus" {
            n113 = global read "Odour_sequences.vi" "Sequences"() -> (w145:T8)
            n114 = property on="Sequences" class="LstBox (strict)"() -> ("Value"=w146:i32)  [unwired: 2 in, 2 out]
            n115 = property on="Stimuli" class="LstBox (strict)"() -> ("Value"=w147:i32)  [unwired: 2 in, 2 out]
            n116 = call "Remove_stimulus.vi"("Value 2"=w147, "Sequences in"=w145, "Value"=w146) -> ("Sequences out"=w144:T8)  [unwired: 8 in]
            n117 = global write "Odour_sequences.vi" "Sequences"(w144) -> ()
            n118 = call "Save_sequences.vi"("Sequences"=w144) -> ()
          }
        }
        n119 = Build Array("Counter bottle", "Stimulus bottle", "Stimulus" ("element"), "Sequence stimulus" ("element")) -> (w127:string[])
        n120 = Search 1D Array(1D array=w127, element=w124) -> (index of element=w125:i32)  [unwired: 1 in]
        n121 = Greater Or Equal To 0?(x=w125) -> (x >= 0?=w126:bool)
        n122 = event-data("Accepted?"=w126) -> ()  [unwired: 1 in, 1 out]
      }
      event "Counter  9-12", "Counter  5-8", "Counter  1-4", "Counter  13-16": Drop {
        n123 = event-data() -> ("CtlRef"=w148:refnum<vi>, "Available Data Names"=w150:string[])  [unwired: 1 in, 7 out]
        n124 = call "Handle_counter_bottle_drop.vi"("Available Data Names"=w150, "ListBox in"=w148) -> ("Boolean"=w149:bool)  [unwired: 9 in]
        n125 = event-data("Accepted?"=w149) -> ()  [unwired: 1 in, 1 out]
      }
      event "Stimulus properties.Add stimulus button": Value Change {
        n126 = event-data() -> ()  [unwired: 1 in, 6 out]
        n127 = property on="Bottles" class="LstBox (strict)"() -> ("Item Names"=w156:string[])  [unwired: 2 in, 2 out]
        n128 = call "Bottle_names_to_bottles.vi"("Item Names"=w156) -> ("Array"=w155:i32[])  [unwired: 10 in]
        n129 = property on="Stimulus properties" class="Clust (strict)"() -> ("Value"=w163:T3)  [unwired: 2 in, 2 out]
        n130 = Unbundle By Name(w163) -> ("Conc."=w162:dbl, "Unit"=w161:enum16{"%", "ppm"}, "Duration"=w160:dbl)  [unwired: 1 out]
        n131 = Bundle By Name(cluster=T9 {"Name"="UNNAMED", "Bottles"=[], "Conc."=1.0, "Unit"=enum."ppm", "Frequency"=250.0} ("Stimulus properties"), "Name"="UNNAMED", "Bottles"=w155, "Conc."=w162, "Unit"=w161, "Frequency"=w160) -> (w158:T9)
        n132 = global read "Odour_stimuli.vi" "Odour stimuli"() -> (w153:T19)
        n133 = Build Array (concatenate)(w153, w158) -> (w152:T7)
        n134 = call "Save_stimuli.vi"("Array"=w152) -> ()
        n135 = global write "Odour_stimuli.vi" "Odour stimuli"(w152) -> ()
        n136 = for {
          tunnel: [w165] -> w157 mode=indexing
          tunnel: w152 -> [w164] mode=indexing
          n137 = Unbundle By Name(w164) -> ("Name"=w165:string)
        }
        n138 = property on="Add stimulus button" class="Bool (strict)"("Value"=FALSE) -> ()  [unwired: 2 in, 2 out]
        n139 = property on="Stimuli" class="LstBox (strict)"("Item Names"=w157) -> ()  [unwired: 2 in, 2 out]
      }
      event "Sequence properties.Add sequence button": Value Change {
        n140 = event-data() -> ()  [unwired: 1 in, 6 out]
        n141 = property on="Stimuli" class="LstBox (strict)"() -> ("Item Names"=w178:string[])  [unwired: 2 in, 2 out]
        n142 = property on="Stimuli" class="LstBox (strict)"() -> ("Item Names"=w179:string[])  [unwired: 2 in, 2 out]
        n143 = for {
          tunnel: w179 -> [w183] mode=indexing
          tunnel: w178 -> [w184]
          tunnel: [w182] -> w176 mode=indexing
          n144 = Search 1D Array(1D array=w184, element=w183) -> (index of element=w182:i32)  [unwired: 1 in]
        }
        n145 = property on="Sequence properties" class="Clust (strict)"() -> ("Value"=w173:T4)  [unwired: 2 in, 2 out]
        n146 = Unbundle By Name(w173) -> ("Trigger"=w171:u16, "Stimulus interval"=w172:dbl, "Reward condition"=w167:u16)  [unwired: 1 out]
        n147 = Bundle By Name(cluster=T10 {"Name"="", "Trigger"=0, "Stimulus interval"=0.0, "Stimuli"=[], "Reward condition"=0} ("Sequences 2"), "Name"="UNNAMED", "Trigger"=w171, "Stimulus interval"=w172, "Reward condition"=w167, "Stimuli"=w176) -> (w175:T10)
        n148 = global read "Odour_sequences.vi" "Sequences"() -> (w177:T8)
        n149 = Build Array (concatenate)(w177, w175) -> (w170:T8)
        n150 = call "Save_sequences.vi"("Sequences"=w170) -> ()
        n151 = global write "Odour_sequences.vi" "Sequences"(w170) -> ()
        n152 = for {
          tunnel: [w181] -> w169 mode=indexing
          tunnel: w170 -> [w180] mode=indexing
          n153 = Unbundle By Name(w180) -> ("Name"=w181:string)
        }
        n154 = property on="Add sequence button" class="Bool (strict)"("Value"=FALSE) -> ()  [unwired: 2 in, 2 out]
        n155 = property on="Sequences" class="LstBox (strict)"("Item Names"=w169) -> ()  [unwired: 2 in, 2 out]
      }
      event "Sequence properties.Remove sequence button": Value Change {
        n156 = event-data() -> ()  [unwired: 1 in, 6 out]
        n157 = global read "Odour_sequences.vi" "Sequences"() -> (w189:T8)
        n158 = property on="Sequences" class="LstBox (strict)"() -> ("Value"=w187:i32)  [unwired: 2 in, 2 out]
        n159 = Delete From Array(array=w189, length=1, index=w187) -> (array with subset deleted=w188:T8)  [unwired: 1 out]
        n160 = global write "Odour_sequences.vi" "Sequences"(w188) -> ()
        n161 = call "Save_sequences.vi"("Sequences"=w188) -> ()
        n162 = property on="Remove sequence button" class="Bool (strict)"("Value"=FALSE) -> ()  [unwired: 2 in, 2 out]
      }
      event "Stimulus properties.Remove stimulus button": Value Change {
        n163 = event-data() -> ()  [unwired: 1 in, 6 out]
        n164 = global read "Odour_stimuli.vi" "Odour stimuli"() -> (w193:T19)
        n165 = property on="Stimuli" class="LstBox (strict)"() -> ("Value"=w194:i32)  [unwired: 2 in, 2 out]
        n166 = Delete From Array(array=w193, length=1, index=w194) -> (array with subset deleted=w192:T19)  [unwired: 1 out]
        n167 = global write "Odour_stimuli.vi" "Odour stimuli"(w192) -> ()
        n168 = call "Save_stimuli.vi"("Array"=w192) -> ()
        n169 = property on="Remove stimulus button" class="Bool (strict)"("Value"=FALSE) -> ()  [unwired: 2 in, 2 out]
      }
      event "Stimuli": Value Change {
        n170 = event-data() -> ("NewVal"=w195:i32)  [unwired: 1 in, 5 out]
        n171 = global read "Odour_stimuli.vi" "Odour stimuli"() -> (w202:T19)
        n172 = Index Array(array=w202, index=w195) -> (element=w201:T20)
        n173 = property on="Stimulus properties" class="Clust (strict)"() -> ("Value"=w208:T3)  [unwired: 2 in, 2 out]
        n174 = Unbundle By Name(w208) -> ("Add stimulus button"=w207:bool, "Remove stimulus button"=w206:bool)
        n175 = Unbundle By Name(w201) -> ("Name"=w199:string, "Bottles"=w200:i32[], "Conc."=w198:dbl, "Unit"=w197:enum16{"%", "ppm"}, "Duration"=w196:dbl)
        n176 = call "Bottles_to_bottle_names.vi"("Bottles"=w200) -> ("Array"=w203:string[])  [unwired: 10 in]
        n177 = Bundle By Name(cluster=w208, "Name"=w199, "Bottles"=0, "Conc."=w198, "Unit"=w197, "Duration"=w196, "Add stimulus button"=w207, "Remove stimulus button"=w206) -> (w205:T3)
        n178 = property on="Stimulus properties" class="Clust (strict)"("Value"=w205) -> ()  [unwired: 2 in, 2 out]
        n179 = property on="Bottles" class="LstBox (strict)"("Item Names"=w203) -> ()  [unwired: 2 in, 2 out]
      }
      event "Sequences": Value Change {
        n180 = event-data() -> ("NewVal"=w221:i32)  [unwired: 1 in, 5 out]
        n181 = global read "Odour_sequences.vi" "Sequences"() -> (w223:T8)
        n182 = property on="Sequence properties" class="Clust (strict)"() -> ("Value"=w213:T4)  [unwired: 2 in, 2 out]
        n183 = Index Array(array=w223, index=w221) -> (element=w222:T10)
        n184 = Unbundle By Name(w213) -> ("Add sequence button"=w212:bool, "Remove sequence button"=w211:bool)
        n185 = Unbundle By Name(w222) -> ("Name"=w216:string, "Trigger"=w215:u16, "Stimulus interval"=w214:dbl, "Reward condition"=w209:u16, "Stimuli"=w219:i32[])
        n186 = property on="Stimuli" class="LstBox (strict)"() -> ("Item Names"=w220:string[])  [unwired: 2 in, 2 out]
        n187 = for {
          tunnel: w220 -> [w226]
          tunnel: w219 -> [w225] mode=indexing
          tunnel: [w224] -> w218 mode=indexing
          n188 = Index Array(array=w226, index=w225) -> (element=w224:string)
        }
        n189 = Bundle By Name(cluster=w213, "Name"=w216, "Trigger"=w215, "Stimulus interval"=w214, "Reward condition"=w209, "Add sequence button"=w212, "Remove sequence button"=w211, "Stimuli"=0) -> (w210:T4)
        n190 = property on="Sequence properties" class="Clust (strict)"("Value"=w210) -> ()  [unwired: 2 in, 2 out]
        n191 = property on="Stimuli" class="LstBox (strict)"("Item Names"=w218) -> ()  [unwired: 2 in, 2 out]
      }
      event Key Down {
        n192 = event-data() -> ("VKey"=w229:T11)  [unwired: 1 in, 9 out]
        n193 = Equal?(x=w229, y=eventvkey."Delete" ("VKey")) -> (x = y?=w227:bool)
        n194 = case shown="False" w227 {
          frame False {
          }
          frame True {
            n195 = property on="Odour bottles" class="Arr (strict)"() -> ("Value"=w232:T5)  [unwired: 2 in, 2 out]
            n196 = call "Empty_bottle.vi"("Odour bottles in"=w232) -> ("Odour bottles out"=w231:T5)  [unwired: 9 in]
            n197 = global read "Odour_component_data_GLOBAL.vi" "Odour component data"() -> (w230:T12)
            n198 = property on="Odour bottles" class="Arr (strict)"("Value"=w231) -> ()  [unwired: 2 in, 2 out]
            n199 = call "Calculate_bottle_distance_matrix.vi"("Odour component data"=w230, "Odour bottles"=w231) -> ("Colour grid"=w233:u32[][])  [unwired: 1 in]
            n200 = property on="DistanceMatrixColorBox" class="Arr (strict)"("Value"=w233) -> ()  [unwired: 2 in, 2 out]
          }
        }
      }
      event "Odour chemicals": Drag Starting? {
        n201 = event-data() -> ("Data"=w238:T21)  [unwired: 1 in, 9 out]
        n202 = global read "Odour_component_data_GLOBAL.vi" "Odour component data"() -> (w234:T12)
        n203 = call "Odour_drag.vi"("Data"=w238, "Odour component data"=w234) -> ("Boolean"=w237:bool, "Data out"=w236:T21)  [unwired: 8 in]
        n204 = event-data("Data"=w236, "Discard?"=w237, "Drag Mode"=enum32{"copy or move", "copy only", "move only"}."copy only") -> ()  [unwired: 1 in, 1 out]
      }
      event "Blank": Drag Starting? {
        n205 = event-data() -> ("Data"=w239:T21)  [unwired: 1 in, 9 out]
        n206 = call "Rename_drag.vi"("data name"="Blank", "Data"=w239) -> ()  [unwired: 9 in, 1 out]
        n207 = event-data("Data"=w239) -> ()  [unwired: 1 in, 1 out]
      }
      event "Counter  5-8", "Counter  9-12", "Counter  1-4", "Counter  13-16": Drag Starting? {
        n208 = event-data() -> ("Data"=w242:T21)  [unwired: 1 in, 9 out]
        n209 = call "Rename_drag.vi"("data name"="Counter bottle", "Data"=w242) -> ("Array"=w241:T21)  [unwired: 9 in]
        n210 = event-data("Data"=w241) -> ()  [unwired: 1 in, 1 out]
      }
      event "Stimuli": Drag Starting? {
        n211 = event-data() -> ("Data"=w245:T21)  [unwired: 1 in, 9 out]
        n212 = call "Rename_drag.vi"("data name"="Stimulus", "Data"=w245) -> ("Array"=w244:T21)  [unwired: 9 in]
        n213 = event-data("Data"=w244) -> ()  [unwired: 1 in, 1 out]
      }
      event "Stimulus properties", "Stimulus properties.Bottles": Value Change {
        n214 = event-data() -> ()  [unwired: 1 in, 6 out]
        n215 = property on="Odour bottles" class="Arr (strict)"() -> ("Value"=w250:T5)  [unwired: 2 in, 2 out]
        n216 = property on="Bottles" class="LstBox (strict)"() -> ("Item Names"=w253:string[])  [unwired: 2 in, 2 out]
        n217 = call "Bottle_names_to_bottles.vi"("Odour bottles"=w250, "Item Names"=w253) -> ("Array"=w252:i32[])  [unwired: 9 in]
        n218 = property on="Stimulus properties" class="Clust (strict)"() -> ("Value"=w260:T3)  [unwired: 2 in, 2 out]
        n219 = Unbundle By Name(w260) -> ("Name"=w259:string, "Conc."=w258:dbl, "Unit"=w257:enum16{"%", "ppm"}, "Duration"=w256:dbl)
        n220 = global read "Odour_stimuli.vi" "Odour stimuli"() -> (w251:T19)
        n221 = Bundle By Name(cluster=T9 {"Name"="", "Bottles"=[], "Conc."=0.0, "Unit"=enum."%", "Frequency"=0.0} ("new element/subarray"), "Name"=w259, "Bottles"=w252, "Conc."=w258, "Unit"=w257, "Frequency"=w256) -> (w254:T9)
        n222 = global read "Odour_component_data_GLOBAL.vi" "Odour component data"() -> (w249:T12)
        n223 = property on="Stimuli" class="LstBox (strict)"() -> ("Value"=w261:i32)  [unwired: 2 in, 2 out]
        n224 = Replace Array Subset(array=w251, new element=w254, index=w261) -> (w247:T19)
        n225 = global write "Odour_stimuli.vi" "Odour stimuli"(w247) -> ()
        n226 = call "Calculate_stimulus_similarity_matrix.vi"("Odour component data"=w249, "Odour bottles"=w250, "Odour stimuli"=w247) -> ("Stimulus similarity"=→"Stimulus similarity":u32[][])
        n227 = call "Save_stimuli.vi"("Array"=w247) -> ()
        n228 = for {
          tunnel: w247 -> [w264] mode=indexing
          tunnel: [w263] -> w262 mode=indexing
          n229 = Unbundle By Name(w264) -> ("Name"=w263:string)
        }
        "Stimulus similarity labels 1" <- w262
        "Stimulus similarity labels 2" <- w262
        n230 = property on="Stimuli" class="LstBox (strict)"("Item Names"=w262) -> ()  [unwired: 2 in, 2 out]
      }
      event "Sequence properties", "Sequence properties.Stimuli": Value Change {
        n231 = event-data() -> ()  [unwired: 1 in, 6 out]
        n232 = property on="Stimuli" class="LstBox (strict)"() -> ("Item Names"=w269:string[])  [unwired: 2 in, 2 out]
        n233 = property on="Stimuli" class="LstBox (strict)"() -> ("Item Names"=w270:string[])  [unwired: 2 in, 2 out]
        n234 = for {
          tunnel: w270 -> [w280] mode=indexing
          tunnel: w269 -> [w281]
          tunnel: [w279] -> w268 mode=indexing
          n235 = Search 1D Array(1D array=w281, element=w280) -> (index of element=w279:i32)  [unwired: 1 in]
        }
        n236 = property on="Sequence properties" class="Clust (strict)"() -> ("Value"=w278:T4)  [unwired: 2 in, 2 out]
        n237 = Unbundle By Name(w278) -> ("Name"=w276:string, "Trigger"=w275:u16, "Stimulus interval"=w274:dbl, "Reward condition"=w266:u16)
        n238 = Bundle By Name(cluster=T10 {"Name"="", "Trigger"=0, "Stimulus interval"=0.0, "Stimuli"=[], "Reward condition"=0} ("Sequences 2"), "Name"=w276, "Trigger"=w275, "Stimulus interval"=w274, "Reward condition"=w266, "Stimuli"=w268) -> (w265:T10)
        n239 = global read "Odour_sequences.vi" "Sequences"() -> (w277:T8)
        n240 = property on="Sequences" class="LstBox (strict)"() -> ("Value"=w273:i32)  [unwired: 2 in, 2 out]
        n241 = Replace Array Subset(array=w277, new element=w265, index=w273) -> (w272:T8)
        n242 = global write "Odour_sequences.vi" "Sequences"(w272) -> ()
        n243 = call "Save_sequences.vi"("Sequences"=w272) -> ()
        n244 = for {
          tunnel: w272 -> [w283] mode=indexing
          tunnel: [w282] -> w271 mode=indexing
          n245 = Unbundle By Name(w283) -> ("Name"=w282:string)
        }
        n246 = property on="Sequences" class="LstBox (strict)"("Item Names"=w271) -> ()  [unwired: 2 in, 2 out]
      }
      event "Sequences": Drag Starting? {
        n247 = event-data() -> ("Data"=w285:T21)  [unwired: 1 in, 9 out]
        n248 = call "Rename_drag.vi"("data name"="Sequence", "Data"=w285) -> ("Array"=w284:T21)  [unwired: 9 in]
        n249 = event-data("Data"=w284) -> ()  [unwired: 1 in, 1 out]
      }
      event "Sequence properties.Stimuli": Drop {
        n250 = event-data() -> ()  [unwired: 1 in, 9 out]
        n251 = Get Drag Drop Data(8:"" ("type"), 9:"Stimulus" ("data name")) -> (0:w287:errorcluster, 3:w289:string)  [unwired: 1 in]
        n252 = call <vilib>:"Clear Errors.vi"("error in (no error)"=w287) -> ()  [unwired: 5 in, 2 out]
        n253 = Unbundle By Name(w287) -> ("status"=w288:bool)
        n254 = case shown="False" w288 {
          tunnel: w289 -> [w293 _]
          frame False {
            n255 = property on="Stimuli" class="LstBox (strict)"() -> ("Item Names"=w294:string[])  [unwired: 2 in, 2 out]
            n256 = Build Array (concatenate)(w294, w293) -> (w292:string[])
            n257 = property on="Stimuli" class="LstBox (strict)"("Item Names"=w292) -> ()  [unwired: 2 in, 2 out]
          }
          frame True {
          }
        }
        n258 = event-data() -> ()  [unwired: 2 in, 1 out]
      }
      event "Protocol cluster.Sequence": Drop {
        n259 = event-data() -> ()  [unwired: 1 in, 9 out]
        n260 = Get Drag Drop Data(8:"" ("type"), 9:"Sequence" ("data name")) -> (0:w299:errorcluster, 3:w297:string)  [unwired: 1 in]
        n261 = call <vilib>:"Clear Errors.vi"("error in (no error)"=w299) -> ()  [unwired: 5 in, 2 out]
        n262 = Unbundle By Name(w299) -> ("status"=w298:bool)
        n263 = case shown="False" w298 {
          tunnel: w297 -> [w308 _]
          tunnel: [w302 errorcluster {"status"=FALSE, "code"=0, "source"=""} ("error out")] -> w296
          frame False {
            n264 = property on="Sequence" class="Arr (strict)"() -> ("Value"=w310:string[])  [unwired: 2 in, 2 out]
            n265 = property on="Rel. requency" class="Arr (strict)"() -> ("Value"=w306:dbl[])  [unwired: 2 in, 2 out]
            n266 = Build Array (concatenate)(w310, w308) -> (w309:string[])
            n267 = property on="Sequence" class="Arr (strict)"("Value"=w309) -> ()  [unwired: 2 in, 2 out]
            n268 = Build Array (concatenate)(w306, 1 ("Numeric")) -> (w304:dbl[])
            n269 = property on="Rel. requency" class="Arr (strict)"("Value"=w304) -> ()  [unwired: 2 in, 2 out]
            n270 = Add Array Elements(numeric array=w304) -> (sum=w307:dbl)
            n271 = Divide(x=w304, y=w307) -> (x/y=w303:dbl[])
            n272 = property on="Frequency" class="Arr (strict)"("Value"=w303) -> (error out=w302:errorcluster)  [unwired: 2 in, 1 out]
          }
          frame True {
          }
        }
        n273 = property on="Protocol cluster" class="Clust (strict)"(error in=w296) -> ("Value"=w295:T2)  [unwired: 1 in, 2 out]
        n274 = global write "Odour_protocol.vi" "Protocol cluster"(w295) -> ()
        n275 = event-data() -> ()  [unwired: 2 in, 1 out]
      }
      event "Clear protocol": Value Change {
        n276 = event-data() -> ()  [unwired: 1 in, 6 out]
        n277 = Two Button Dialog(message="Are you sure you want to clear all protocol data?", 2:"Clear" ("T button name (\"OK\")")) -> (T button?=w312:bool)  [unwired: 1 in]
        n278 = case shown="True" w312 {
          frame False {
          }
          frame True {
            w315 = T2 {"Sequence"=[], "Rel. requency"=[], "Frequency"=[], "Sequence interval"=200.0, "Rarest sequence "=200.0, "Randomization"=0} ("Protocol cluster")
            n279 = property on="Clear protocol" class="Bool (strict)"("Value"=FALSE ("Clear protocol")) -> ()  [unwired: 2 in, 2 out]
            n280 = global write "Odour_protocol.vi" "Protocol cluster"(w315) -> ()
            n281 = property on="Protocol cluster" class="Clust (strict)"("Value"=w315) -> ()  [unwired: 2 in, 2 out]
          }
        }
      }
      event "Protocol cluster.Rel. requency": Value Change {
        n282 = event-data() -> ()  [unwired: 1 in, 6 out]
        n283 = property on="Rel. requency" class="Arr (strict)"() -> ("Value"=w323:dbl[])  [unwired: 2 in, 2 out]
        n284 = Add Array Elements(numeric array=w323) -> (sum=w324:dbl)
        n285 = property on="Sequence interval" class="DigNum (strict)"() -> ("Value"=w321:dbl)  [unwired: 2 in, 2 out]
        n286 = Divide(x=w323, y=w324) -> (x/y=w319:dbl[])
        n287 = property on="Frequency" class="Arr (strict)"("Value"=w319) -> ()  [unwired: 2 in, 2 out]
        n288 = Divide(x=3600000.0, y=w321) -> (x/y=w320:dbl)
        n289 = Array Max & Min(array=w319) -> (min value=w318:dbl)  [unwired: 3 out]
        n290 = Multiply(x=w320, y=w318) -> (x*y=w317:dbl)
        n291 = property on="Rarest sequence" class="DigNum (strict)"("Value"=w317) -> ()  [unwired: 2 in, 2 out]
      }
      event "Protocol": Value Change {
        n292 = event-data() -> ("NewVal"=w328:path)  [unwired: 1 in, 5 out]
        n293 = call <vilib>:"Check if File or Folder Exists.vi"("path"=w328) -> ("error out"=w325:errorcluster, "file or folder exists?"=w327:bool, "dup path"=w326:path)  [unwired: 8 in]
        n294 = case shown="False" w327 {
          tunnel: w326 -> [_ w334]
          tunnel: w325 -> [_ w333]
          frame False {
            w329 = T2 {"Sequence"=[], "Rel. requency"=[], "Frequency"=[], "Sequence interval"=200.0, "Rarest sequence "=200.0, "Randomization"=0} ("Protocol cluster")
            n295 = global write "Odour_protocol.vi" "Protocol cluster"(w329) -> ()
            n296 = property on="Protocol cluster" class="Clust (strict)"("Value"=w329) -> ()  [unwired: 2 in, 2 out]
          }
          frame True {
            n297 = call-poly <vilib>:"Read From XML File.vi"("error in (no error)"=w333, "XML File Path"=w334) -> ("error out"=w331:errorcluster, "XML Elements"=w332:string)  [unwired: 7 in, 1 out]
            n298 = call "Load_protocol.vi"("error in (no error)"=w331, "XML Elements"=w332) -> ("Protocol cluster"=w330:T2)  [unwired: 8 in, 1 out]
            n299 = global write "Odour_protocol.vi" "Protocol cluster"(w330) -> ()
            n300 = property on="Protocol cluster" class="Clust (strict)"("Value"=w330) -> ()  [unwired: 2 in, 2 out]
          }
        }
      }
      event "Save protocol": Value Change {
        n301 = event-data() -> ()  [unwired: 1 in, 6 out]
        n302 = property on="Randomization" class="Ring (strict)" props=["Value"]() -> ()  [unwired: 2 in, 3 out]
        n303 = call <vilib>:"Check if File or Folder Exists.vi"("path"="Protocol") -> ("file or folder exists?"=w337:bool)  [unwired: 8 in, 2 out]
        n304 = case shown="True" w337 {
          tunnel: [TRUE ("T button?") w341] -> w336
          frame False {
          }
          frame True {
            n305 = Two Button Dialog(message="File exists. Are you sure you want to overwrite it?", 1:"No" ("F button name (\"Cancel\")"), 2:"Yes" ("T button name (\"OK\")")) -> (T button?=w341:bool)
          }
        }
        n306 = case shown="True" w336 {
          tunnel: "Protocol" -> [_ w338]
          frame False {
          }
          frame True {
            n307 = global read "Odour_protocol.vi" "Protocol cluster"() -> (w339:T2)
            n308 = call "Save_protocol.vi"("Protocol cluster"=w339, "Protocol File Path"=w338) -> ()  [unwired: 1 in]
          }
        }
      }
      event "Stimulus properties.Bottles": Drag Starting? {
        n309 = event-data() -> ("Data"=w346:T21)  [unwired: 1 in, 9 out]
        n310 = call "Rename_drag.vi"("data name"="Stimulus bottle", "Data"=w346) -> ("Array"=w345:T21)  [unwired: 9 in]
        n311 = event-data("Data"=w345) -> ()  [unwired: 1 in, 1 out]
      }
      event "Sequence properties.Stimuli": Drag Starting? {
        n312 = event-data() -> ("Data"=w349:T21)  [unwired: 1 in, 9 out]
        n313 = call "Rename_drag.vi"("data name"="Sequence stimulus", "Data"=w349) -> ("Array"=w348:T21)  [unwired: 9 in]
        n314 = event-data("Data"=w348) -> ()  [unwired: 1 in, 1 out]
      }
    }
  }
